vi "NEO Set Pod Setpoints.vi"(6 "Operation":T4, 8 "Steer Angles (degrees)":T5, 9 "Drive Velocities (ft/s)":T5, 10 "Pod Setpoints (ft/s and deg)":T17, 11 "Swerve Drive":T6={"Drive Motors (NEO)"={"Left Front"={"DeviceStatus"={"status"=FALSE, "code"=0, "source"=""}, "Type"=enum."PWM", "PWM"={"PWM Channel"=enum."Invalid", "DeadBand"={"Name"="", "maxPositivePwm"=0, "minPositivePwm"=0, "centerPwm"=0, "maxNegativePwm"=0, "minNegativePwm"=0, "angularRange"=0}}, "CAN"={"Device Number"=0, "SetOutput VI Ref"=variant, "GetOutput VI Ref"=variant, "Enable VI Ref"=variant, "Disable VI Ref"=variant, "Data"=variant}, "Invert"=FALSE, "DIO PWM"={"PWM \"Enable\" Channel"=enum."Invalid", "DIOChannel"=enum."Invalid", "PWM Rate"=0.0}}, "Left Back"={"DeviceStatus"={"status"=FALSE, "code"=0, "source"=""}, "Type"=enum."PWM", "PWM"={"PWM Channel"=enum."Invalid", "DeadBand"={"Name"="", "maxPositivePwm"=0, "minPositivePwm"=0, "centerPwm"=0, "maxNegativePwm"=0, "minNegativePwm"=0, "angularRange"=0}}, "CAN"={"Device Number"=0, "SetOutput VI Ref"=variant, "GetOutput VI Ref"=variant, "Enable VI Ref"=variant, "Disable VI Ref"=variant, "Data"=variant}, "Invert"=FALSE, "DIO PWM"={"PWM \"Enable\" Channel"=enum."Invalid", "DIOChannel"=enum."Invalid", "PWM Rate"=0.0}}, "Right Front"={"DeviceStatus"={"status"=FALSE, "code"=0, "source"=""}, "Type"=enum."PWM", "PWM"={"PWM Channel"=enum."Invalid", "DeadBand"={"Name"="", "maxPositivePwm"=0, "minPositivePwm"=0, "centerPwm"=0, "maxNegativePwm"=0, "minNegativePwm"=0, "angularRange"=0}}, "CAN"={"Device Number"=0, "SetOutput VI Ref"=variant, "GetOutput VI Ref"=variant, "Enable VI Ref"=variant, "Disable VI Ref"=variant, "Data"=variant}, "Invert"=FALSE, "DIO PWM"={"PWM \"Enable\" Channel"=enum."Invalid", "DIOChannel"=enum."Invalid", "PWM Rate"=0.0}}, "Right Back"={"DeviceStatus"={"status"=FALSE, "code"=0, "source"=""}, "Type"=enum."PWM", "PWM"={"PWM Channel"=enum."Invalid", "DeadBand"={"Name"="", "maxPositivePwm"=0, "minPositivePwm"=0, "centerPwm"=0, "maxNegativePwm"=0, "minNegativePwm"=0, "angularRange"=0}}, "CAN"={"Device Number"=0, "SetOutput VI Ref"=variant, "GetOutput VI Ref"=variant, "Enable VI Ref"=variant, "Disable VI Ref"=variant, "Data"=variant}, "Invert"=FALSE, "DIO PWM"={"PWM \"Enable\" Channel"=enum."Invalid", "DIOChannel"=enum."Invalid", "PWM Rate"=0.0}}}, "Steer Motors (NEO)"={"Left Front"={"DeviceStatus"={"status"=FALSE, "code"=0, "source"=""}, "Type"=enum."PWM", "PWM"={"PWM Channel"=enum."Invalid", "DeadBand"={"Name"="", "maxPositivePwm"=0, "minPositivePwm"=0, "centerPwm"=0, "maxNegativePwm"=0, "minNegativePwm"=0, "angularRange"=0}}, "CAN"={"Device Number"=0, "SetOutput VI Ref"=variant, "GetOutput VI Ref"=variant, "Enable VI Ref"=variant, "Disable VI Ref"=variant, "Data"=variant}, "Invert"=FALSE, "DIO PWM"={"PWM \"Enable\" Channel"=enum."Invalid", "DIOChannel"=enum."Invalid", "PWM Rate"=0.0}}, "Left Back"={"DeviceStatus"={"status"=FALSE, "code"=0, "source"=""}, "Type"=enum."PWM", "PWM"={"PWM Channel"=enum."Invalid", "DeadBand"={"Name"="", "maxPositivePwm"=0, "minPositivePwm"=0, "centerPwm"=0, "maxNegativePwm"=0, "minNegativePwm"=0, "angularRange"=0}}, "CAN"={"Device Number"=0, "SetOutput VI Ref"=variant, "GetOutput VI Ref"=variant, "Enable VI Ref"=variant, "Disable VI Ref"=variant, "Data"=variant}, "Invert"=FALSE, "DIO PWM"={"PWM \"Enable\" Channel"=enum."Invalid", "DIOChannel"=enum."Invalid", "PWM Rate"=0.0}}, "Right Front"={"DeviceStatus"={"status"=FALSE, "code"=0, "source"=""}, "Type"=enum."PWM", "PWM"={"PWM Channel"=enum."Invalid", "DeadBand"={"Name"="", "maxPositivePwm"=0, "minPositivePwm"=0, "centerPwm"=0, "maxNegativePwm"=0, "minNegativePwm"=0, "angularRange"=0}}, "CAN"={"Device Number"=0, "SetOutput VI Ref"=variant, "GetOutput VI Ref"=variant, "Enable VI Ref"=variant, "Disable VI Ref"=variant, "Data"=variant}, "Invert"=FALSE, "DIO PWM"={"PWM \"Enable\" Channel"=enum."Invalid", "DIOChannel"=enum."Invalid", "PWM Rate"=0.0}}, "Right Back"={"DeviceStatus"={"status"=FALSE, "code"=0, "source"=""}, "Type"=enum."PWM", "PWM"={"PWM Channel"=enum."Invalid", "DeadBand"={"Name"="", "maxPositivePwm"=0, "minPositivePwm"=0, "centerPwm"=0, "maxNegativePwm"=0, "minNegativePwm"=0, "angularRange"=0}}, "CAN"={"Device Number"=0, "SetOutput VI Ref"=variant, "GetOutput VI Ref"=variant, "Enable VI Ref"=variant, "Disable VI Ref"=variant, "Data"=variant}, "Invert"=FALSE, "DIO PWM"={"PWM \"Enable\" Channel"=enum."Invalid", "DIOChannel"=enum."Invalid", "PWM Rate"=0.0}}}, "PigeonIMUDevRef"={"DeviceStatus"={"status"=FALSE, "code"=0, "source"=""}, "Device Number"=0, "Type"=352321536, "Device ID"=0, "Handle"=0, "UsageFrame"=0, "Library Path"=path ""}, "Radii (ft)"={"Left Front Position"=[], "Left Back Position"=[], "Right Front Position"=[], "Right Back Position"=[]}} {"PigeonIMUDevRef"."Type" items=["CAN"=352321536, "TalonSRX"=33554432]; "Radii (ft)"."Right Back Position" format="%.2f"; "Radii (ft)"."Right Front Position" format="%.2f"; "Radii (ft)"."Left Back Position" format="%.2f"; "Radii (ft)"."Left Front Position" format="%.2f"}) -> ()   [LabVIEW 2025]
uses:
  Type Definitions/Data/Pod Setpoints.ctl
  Type Definitions/Hardware/Swerve Drives/(NEO-NEO-ThroughBore-Pigeon2) Swerve.ctl
  Type Definitions/Hardware/4 Motor Sets/(NEO & NEO 550) 4 Motor Set.ctl
  <vilib>/Rock Robotics/WPI/MotorControl/WPI_MotorControlDeviceRef.ctl
  <vilib>/Rock Robotics/WPI/MotorControl/WPI_MotorControlType.ctl
  <vilib>/Rock Robotics/SystemInterfaces/DIO/FPGA_DIOPWMChannel.ctl
  <vilib>/Rock Robotics/WPI/PWM/WPI_PWMDeadband.ctl
  <vilib>/Rock Robotics/SystemInterfaces/DIO/FPGA_DIOChannel.ctl
  <vilib>/Rock Robotics/WPI/ThirdParty/Phoenix-LabVIEW/Pigeon IMU/CTRE_PigeonIMU_DeviceRef.ctl
  <vilib>/Rock Robotics/WPI/ThirdParty/Phoenix-LabVIEW/Pigeon IMU/CTRE_PigeonIMU_ConnectionType.ctl
  Type Definitions/Data/Pod Positions.ctl
  Robot Code/Drive/Implementation/Drive Operations.ctl
  <vilib>/Rock Robotics/WPI/ThirdParty/REV Robotics/REVLib/Typedef/SPARK Feed Forward Gains.ctl
  <vilib>/Rock Robotics/WPI/ThirdParty/REV Robotics/REVLib/Typedef/Spark MAX Control Type.ctl
  4b768f86-8279-4062-bf26-12cbbaf62c6c.vi
panel:
  in  "Drive PID Gains":T2
  out "Arbitrary":T3
  in  "Motor Type":enum16{"Drive", "Steer"}(ring)
  in  "Motor Position":T16(ring)
  out "PID Graph":cluster{"Left Front":dbl, "Theta":dbl}(graph)
  out "Values":cluster{"Actual":dbl, "Setpoint":dbl}
  in  "Debug Mode?":bool
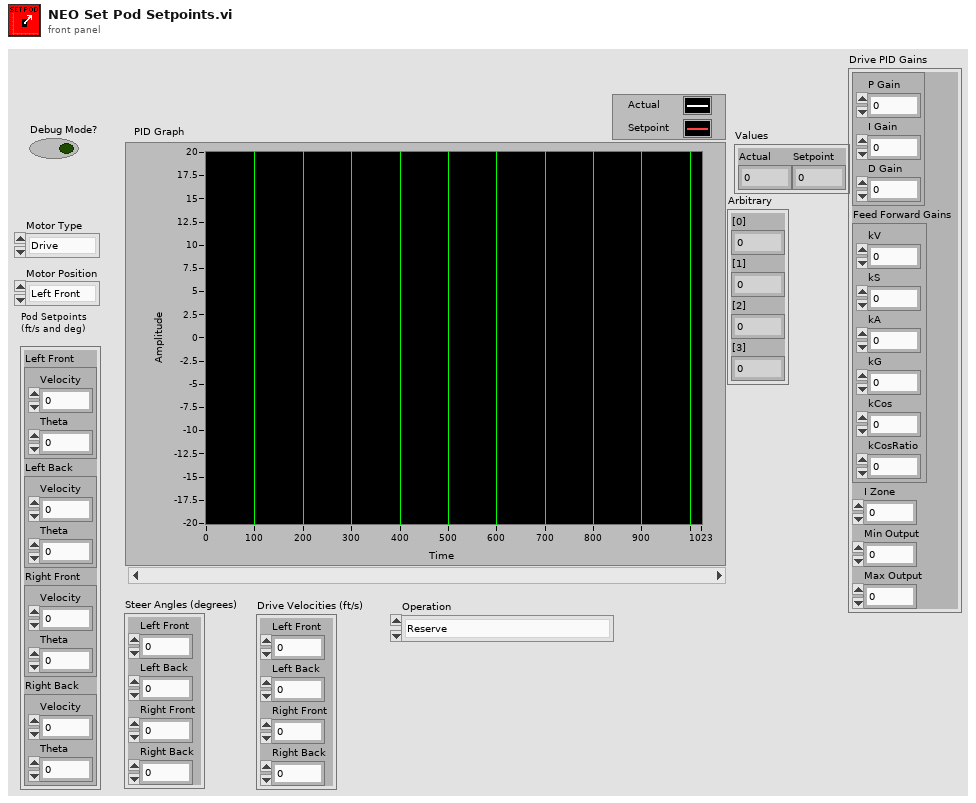
[diagram p1: front panel]
types:
  T1 = typedef "SPARK Feed Forward Gains.ctl" = cluster{"kV":dbl, "kS":dbl, "kA":dbl, "kG":dbl, "kCos":dbl, "kCosRatio":dbl}
  T2 = cluster{cluster{"P Gain":dbl, "I Gain":dbl, "D Gain":dbl}, "Feed Forward Gains":T1, "I Zone":dbl, "Min Output":dbl, "Max Output":dbl}
  T3 = cluster{"[0]":dbl, "[1]":dbl, "[2]":dbl, "[3]":dbl}
  T4 = typedef "Drive Operations.ctl" = enum16{"Reserve", "Read Current", "Immediate", "Calibrate", "Auto", "Auto Pickup"}
  T5 = cluster{"Left Front":dbl, "Left Back":dbl, "Right Front":dbl, "Right Back":dbl}
  T6 = typedef "(NEO-NEO-ThroughBore-Pigeon2) Swerve.ctl" = cluster{"Drive Motors (NEO)":T7, "Steer Motors (NEO)":T7, "PigeonIMUDevRef":T13, "Radii (ft)":T15}
  T7 = typedef "(NEO & NEO 550) 4 Motor Set.ctl" = cluster{"Left Front":T8, "Left Back":T8, "Right Front":T8, "Right Back":T8}
  T8 = typedef "WPI_MotorControlDeviceRef.ctl" = cluster{"DeviceStatus":errorcluster, "Type":T9, "PWM":cluster{"PWM Channel":T10, "DeadBand":T11}, "CAN":cluster{"Device Number":u8, "SetOutput VI Ref":variant, "GetOutput VI Ref":variant, "Enable VI Ref":variant, "Disable VI Ref":variant, "Data":variant}, "Invert":bool, "DIO PWM":cluster{"PWM \"Enable\" Channel":T10, "DIOChannel":T12, "PWM Rate":dbl}}
  T9 = typedef "WPI_MotorControlType.ctl" = enum16{"PWM", "CAN", "DIO PWM"}
  T10 = typedef "FPGA_DIOPWMChannel.ctl" = enum8{"PWM 0", "PWM 1", "PWM 2", "PWM 3", "PWM 4", "PWM 5", "PWM 6", "PWM 7", "PWM 8", "PWM 9", "PWM MXP 0", "PWM MXP 1", "PWM MXP 2", "PWM MXP 3", "PWM MXP 4", "PWM MXP 5", "PWM MXP 6", "PWM MXP 7", "PWM MXP 8", "PWM MXP 9", "Invalid"}
  T11 = typedef "WPI_PWMDeadband.ctl" = cluster{"Name":string, "maxPositivePwm":i32, "minPositivePwm":i32, "centerPwm":i32, "maxNegativePwm":i32, "minNegativePwm":i32, "angularRange":u16}
  T12 = typedef "FPGA_DIOChannel.ctl" = enum8{"DIO 0", "DIO 1", "DIO 2", "DIO 3", "DIO 4", "DIO 5", "DIO 6", "DIO 7", "DIO 8", "DIO 9", "DIO MXP 0", "DIO MXP 1", "DIO MXP 2", "DIO MXP 3", "DIO MXP 4", "DIO MXP 5", "DIO MXP 6", "DIO MXP 7", "DIO MXP 8", "DIO MXP 9", "DIO MXP 10", "DIO MXP 11", "DIO MXP 12", "DIO MXP 13", "DIO MXP 14", "DIO MXP 15", "SPI Port CS1", "SPI Port CS2", "SPI Port CS3", "SPI Port MISO", "SPI Port MOSI", "Invalid"}
  T13 = typedef "CTRE_PigeonIMU_DeviceRef.ctl" = cluster{"DeviceStatus":errorcluster, "Device Number":u8, "Type":T14, "Device ID":u32, "Handle":u64, "UsageFrame":u32, "Library Path":path}
  T14 = typedef "CTRE_PigeonIMU_ConnectionType.ctl" = u32
  T15 = typedef "Pod Positions.ctl" = cluster{"Left Front Position":dbl[], "Left Back Position":dbl[], "Right Front Position":dbl[], "Right Back Position":dbl[]}
  T16 = enum16{"Left Front", "Left Back", "Right Front", "Right Back"}
  T17 = typedef "Pod Setpoints.ctl" = cluster{"Left Front":cluster{"Velocity":dbl, "Theta":dbl}, "Left Back":cluster{"Velocity":dbl, "Theta":dbl}, "Right Front":cluster{"Velocity":dbl, "Theta":dbl}, "Right Back":cluster{"Velocity":dbl, "Theta":dbl}}
  T18 = typedef "Spark MAX Control Type.ctl" = enum16{"Percent VBus", "Voltage", "Velocity", "Position", "Smart Motion", "Current", "Smart Velocity", "MAXMotion Position", "MAXMotion Velocity"}
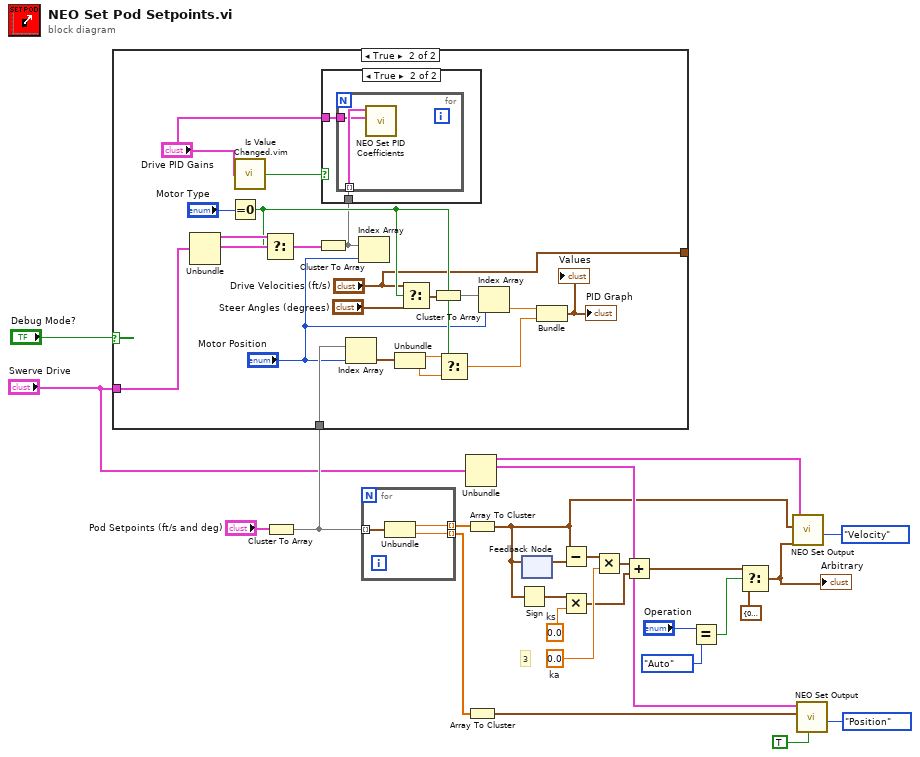
[diagram p0: block diagram]
diagram:
  w16 = 0.0  # ks
  w19 = 0.0  # ka
  # "3"
  n1 = Cluster To Array(cluster="Pod Setpoints (ft/s and deg)") -> (array=w24:cluster{"Velocity":dbl, "Theta":dbl}[])
  n2 = case shown="True" "Debug Mode?" {
    tunnel: "Swerve Drive" -> [_ w34]
    tunnel: w24 -> [_ w35]
    tunnel: [_ "Drive Velocities (ft/s)"] -> _
    frame False {
    }
    frame True {
      n3 = Unbundle(w34) -> ("Drive Motors (NEO)"=w46:T7, "Steer Motors (NEO)"=w45:T7)  [unwired: 2 out]
      n4 = Equal To 0?(x="Motor Type") -> (x = 0?=w40:bool)
      n5 = call "Is Value Changed.vim"("value"="Drive PID Gains") -> ("changed or first call?"=w29:bool)
      n6 = Select(t=w46, s=w40, f=w45) -> (s? t:f=w33:T7)
      n7 = Cluster To Array(cluster=w33) -> (array=w28:T8[])
      n8 = case shown="True" w29 {
        tunnel: w28 -> [_ w49]
        tunnel: "Drive PID Gains" -> [_ w48]
        frame False {
        }
        frame True {
          n9 = for {
            tunnel: w49 -> [w51] mode=indexing
            tunnel: w48 -> [w50]
            n10 = call "NEO Set PID Coefficients.vi"("Drive PID Gains"=w50, "MotorControlDeviceRef in"=w51) -> ()  [unwired: 6 in, 2 out]
          }
        }
      }
      n11 = Index Array(array=w35, index="Motor Position") -> (element=w44:cluster{"Velocity":dbl, "Theta":dbl})
      n12 = Index Array(array=w28, index="Motor Position") -> ()  [unwired: 1 out]
      n13 = Unbundle(w44) -> ("Velocity"=w43:dbl, "Theta"=w42:dbl)
      n14 = Select(t="Drive Velocities (ft/s)", s=w40, f="Steer Angles (degrees)") -> (s? t:f=w39:T5)
      n15 = Cluster To Array(cluster=w39) -> (array=w38:dbl[])
      n16 = Select(t=w43, s=w40, f=w42) -> (s? t:f=w36:dbl)
      n17 = Index Array(array=w38, index="Motor Position") -> (element=w37:dbl)
      n18 = Bundle("Left Front"=w37, "Theta"=w36) -> (→"PID Graph" →"Values":cluster{"Left Front":dbl, "Theta":dbl})  [unwired: 1 in]
    }
  }
  n19 = for {
    tunnel: w24 -> [w54] mode=indexing
    tunnel: [w53] -> w23 mode=indexing
    tunnel: [w52] -> w22 mode=indexing
    n20 = Unbundle(w54) -> ("Velocity"=w53:dbl, "Theta"=w52:dbl)
  }
  n21 = Unbundle("Swerve Drive") -> ("Drive Motors (NEO)"=w21:T7, "Steer Motors (NEO)"=w14:T7)  [unwired: 2 out]
  n22 = Array To Cluster(array=w23) -> (cluster=w4:T3)
  n23 = Array To Cluster(array=w22) -> (cluster=w5:T3)
  n24 = Sign(1:w4) -> (0:w17:T3)
  n25 = feedback #1() -> (w20:T3)  [unwired: 1 in]
  n26 = feedback-in #1(w4) -> ()
  n27 = Subtract(x=w4, y=w20) -> (x-y=w13:T3)
  n28 = Multiply(x=w17, y=w16) -> (x*y=w15:T3)
  n29 = Multiply(x=w13, y=w19) -> (x*y=w18:T3)
  n30 = Add(x=w18, y=w15) -> (x+y=w11:T3)
  n31 = Equal?(x="Operation", y=Drive_Operations."Auto") -> (x = y?=w6:bool)
  n32 = Select(t=w11, s=w6, f=T3 {"[0]"=0.0, "[1]"=0.0, "[2]"=0.0, "[3]"=0.0}) -> (s? t:f=w8:T3)
  "Arbitrary" <- w8
  n33 = call "NEO Set Output.vi"("Arbitrary Feedforward"=w8, "Control Mode"=Spark_MAX_Control_Type."Velocity", "Setpoints"=w4, "Motors"=w21) -> ()  [unwired: 8 in]
  n34 = call "NEO Set Output.vi"("Add Angle Offsets?"=TRUE, "Control Mode"=Spark_MAX_Control_Type."Position", "Setpoints"=w5, "Motors"=w14) -> ()  [unwired: 8 in]
